vi "Init.vi"(8 "error in (no error)":errorcluster, 11 "Coca Actor in":refnum<class "Coca Actor.lvclass">) -> (0 "error out":errorcluster, 3 "Coca Actor out":refnum<class "Coca Actor.lvclass">)   [LabVIEW 2020, in "Coca Actor.lvlib" / "Coca Actor.lvclass"]
uses:
  Coca Actor.lvclass
  Coca Actor.lvclass/Coca Actor.ctl
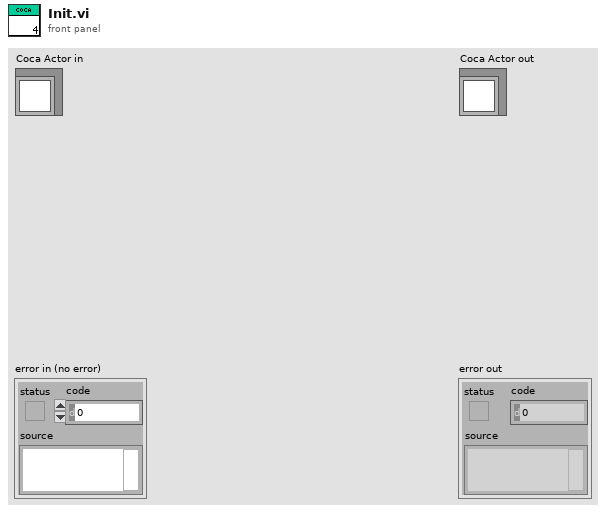
[diagram p1: front panel]
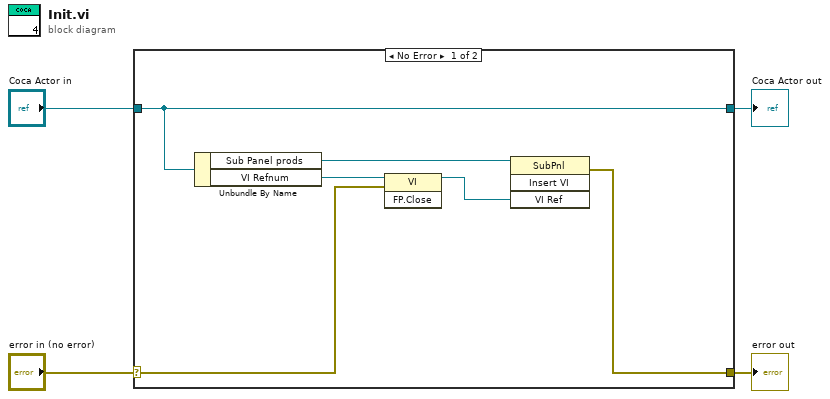
[diagram p0: block diagram]
diagram:
  n1 = case shown="No Error" "error in (no error)" {
    selector: "error in (no error)" -> [w6 w12]
    tunnel: [w5 w12] -> w3
    tunnel: [w7 w11] -> w1
    tunnel: "Coca Actor in" -> [w7 w11]
    frame No Error {
      n2 = Unbundle By Name(w7) -> ("Sub Panel prods"=w8:refnum<vi>, "VI Refnum"=w9:refnum<vi>)
      n3 = invoke class="VI" method="FP.Close"(reference=w9, error in=w6) -> (reference out=w10:refnum<vi>)  [unwired: 1 in, 2 out]
      n4 = invoke class="SubPnl" method="Insert VI"(reference=w8, "VI Ref"=w10) -> (error out=w5:errorcluster)  [unwired: 2 in, 3 out]
    }
    frame Error {
    }
  }
  "error out" <- w3
  "Coca Actor out" <- w1
